vi "WriteDispenseCount (SubVI).vi"(10 "Base Path":path, 11 "Array of UInt16":u16[](array[numeric])) -> ()   [LabVIEW 2013]
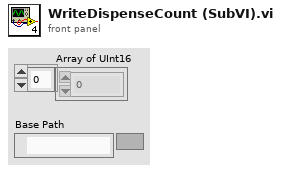
[diagram p1: front panel]
types:
  T1 = enum16{"open", "replace", "create", "open or create", "replace or create", "replace or create with confirmation"}
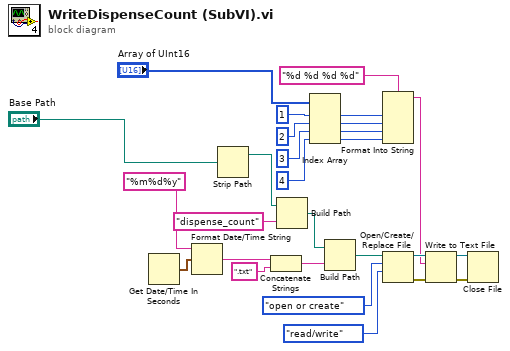
[diagram p0: block diagram]
diagram:
  n1 = Get Date/Time In Seconds() -> (seconds since 1Jan1904=w20:timestamp)
  n2 = Format Date/Time String(time format string (%c)="%m%d%y", seconds (now)=w20) -> (date/time string=w18:string)  [unwired: 1 in]
  n3 = Strip Path(path="Base Path") -> (stripped path=w12:path)  [unwired: 1 out]
  n4 = Concatenate Strings(w18, ".txt" ("string")) -> (w16:string)
  n5 = Build Path(base path=w12, name or relative path="dispense_count") -> (appended path=w21:path)
  n6 = Index Array(array="Array of UInt16", index #1=1 ("index"), index #2=2 ("index"), index #3=3 ("index"), index #4=4 ("index")) -> (element #1=w6:u16, element #2=w7:u16, element #3=w8:u16, element #4=w9:u16)
  n7 = Build Path(base path=w21, name or relative path=w16) -> (appended path=w22:path)
  n8 = Format Into String(format string="%d %d %d %d", w6, w7, w8, w9) -> (resulting string=w25:string)  [unwired: 2 in, 1 out]
  n9 = Open/Create/Replace File(file path (use dialog)=w22, operation (0:open)=T1."open or create", access (0:read/write)=enum16{"read/write", "read-only", "write-only"}."read/write") -> (refnum out=w26:refnum<file>, error out=w14:errorcluster)  [unwired: 3 in, 1 out]
  n10 = Write to Text File(file (use dialog)=w26, text=w25, error in=w14) -> (refnum out=w27:refnum<file>, error out=w15:errorcluster)  [unwired: 1 in, 1 out]
  n11 = Close File(refnum=w27, error in=w15) -> ()  [unwired: 2 out]
